vi "REPORT_OKNOK_save_pdf.vi"(8 "error_in":errorcluster) -> (0 "error_out":errorcluster)   [LabVIEW 2019]
uses:
  FGV/REPORTS_records_display/FGV_REPORTS_records_display.ctl
  typedef/REPORT_OKNOK_all_info.ctl
  <vilib>/Exaprom PDF/Controls/Table Controls/Row Predefined borders cluster.ctl
  <vilib>/Exaprom PDF/Controls/Table Controls/Row Predefined borders.ctl
  <vilib>/Exaprom PDF/Controls/Page Controls/Page setup.ctl
  <vilib>/Exaprom PDF/Controls/Page Controls/Page size.ctl
  <vilib>/Exaprom PDF/Controls/Page Controls/Page Orientation.ctl
  <vilib>/Exaprom PDF/Controls/Page Controls/Page Layout Custom.ctl
  <vilib>/Exaprom PDF/Controls/Page Controls/Page margins.ctl
  REPORT_font_for_pdf_report.ctl
  <vilib>/Exaprom PDF/Controls/Font Controls/Font size.ctl
  <vilib>/Exaprom PDF/Controls/Font Controls/Font color.ctl
  <vilib>/Exaprom PDF/Controls/Font Controls/Type and encoding.ctl
  <vilib>/Exaprom PDF/Controls/Text Controls/Unicode/Type and run direction.ctl
  <vilib>/Exaprom PDF/Controls/Table Controls/Cell Font, type, Alignment and LS V2.ctl
  <vilib>/Exaprom PDF/Controls/Table Controls/Cell Type, Alignment and LS.ctl
  <vilib>/Exaprom PDF/Controls/Table Controls/Cell Alignment 20px.ctl
  <vilib>/Exaprom PDF/Controls/Table Controls/Text vertical arrangement.ctl
  <vilib>/Exaprom PDF/Controls/Text Controls/Line spacing.ctl
  <vilib>/Exaprom PDF/Controls/Font Controls/Font complete cluster.ctl
  <vilib>/Exaprom PDF/Controls/Image Controls/Image alignment and position.ctl
  <vilib>/Exaprom PDF/Controls/Image Controls/Image aligment.ctl
  <vilib>/Exaprom PDF/Controls/Table Controls/Table properties.ctl
  <vilib>/Exaprom PDF/Controls/Table Controls/Table position.ctl
  _misc/AULocalize/SubVIs/Get Localized Phrase Compact Interface 0D.vi
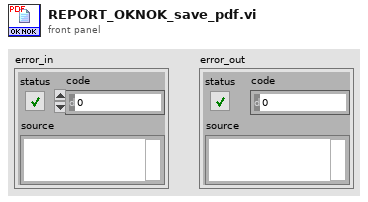
[diagram p1: front panel]
types:
  T1 = typedef "REPORT_OKNOK_all_info.ctl" = cluster{"date_start":string, "date_end":string, "time_start":string, "time_end":string, "records":string[][], "column_headers":string[], "column_widths":i16[]}
  T2 = typedef "FGV_REPORTS_records_display.ctl" = enum16{"initialize", "GEAR_set_serial", "GEAR_set_header", "GEAR_set_operations", "GEAR_set_results", "GEAR_set_batches", "GEAR_get_serial", "GEAR_get_operation_IDs", "GEAR_toggle_results", "GEAR_show_all_results", "GEAR_hide_all_results", "GEAR_display", "GEAR_filter", "GEAR_restore", "GEAR_clear", "GEAR_get_all_info", "DATES_set_dates", "DATES_set_gears", "DATES_display", "DATES_filter", "DATES_first_page", "DATES_previous_page", "DATES_next_page", "DATES_last_page", "DATES_restore", "DATES_clear", "DATES_get_all_info", "PBATCH_set_batch_no", "PBATCH_set_gears", "PBATCH_display", "PBATCH_filter", "PBATCH_first_page", "PBATCH_previous_page", "PBATCH_next_page", "PBATCH_last_page", "PBATCH_restore", "PBATCH_clear", "PBATCH_get_all_info", "OPRTN_set_OP", "OPRTN_set_dates", "OPRTN_set_gears", "OPRTN_set_hidden_columns", "OPRTN_display", "OPRTN_filter", "OPRTN_filter_no_page_reset", "OPRTN_first_page", "OPRTN_previous_page", "OPRTN_next_page", "OPRTN_last_page", "OPRTN_restore", "OPRTN_clear", "OPRTN_get_all_info", "CFG_set_type", "CFG_set_dates", "CFG_set_records", "CFG_display", "CFG_filter", "CFG_first_page", "CFG_previous_page", "CFG_next_page", "CFG_last_page", "CFG_restore", "CFG_clear", "CFG_get_all_info", "AUDIT_set_dates", "AUDIT_set_records", "AUDIT_display", "AUDIT_filter", "AUDIT_first_page", "AUDIT_previous_page", "AUDIT_next_page", "AUDIT_last_page", "AUDIT_restore", "AUDIT_clear", "AUDIT_get_all_info", "OKNOK_set_dates", "OKNOK_set_records", "OKNOK_display", "OKNOK_restore", "OKNOK_clear", "OKNOK_get_all_info", "REWORKS_set_dates", "REWORKS_set_from_to", "REWORKS_set_records", "REWORKS_display", "REWORKS_filter", "REWORKS_first_page", "REWORKS_previous_page", "REWORKS_next_page", "REWORKS_last_page", "REWORKS_restore", "REWORKS_clear", "REWORKS_get_all_info", "PACE_set_dates", "PACE_set_limits", "PACE_set_records", "PACE_display", "PACE_restore", "PACE_clear", "PACE_get_all_info", "CBATCH_set_code", "CBATCH_set_records", "CBATCH_display", "CBATCH_filter", "CBATCH_first_page", "CBATCH_previous_page", "CBATCH_next_page", "CBATCH_last_page", "CBATCH_restore", "CBATCH_clear", "CBATCH_get_all_info", "CMPNT_set_serial", "CMPNT_set_records", "CMPNT_display", "CMPNT_first_page", "CMPNT_previous_page", "CMPNT_next_page", "CMPNT_last_page", "CMPNT_restore", "CMPNT_clear", "CMPNT_get_all_info", "clear"}
  T3 = typedef "Table properties.ctl" = cluster{"Table position":T4, "SpacingBefore (points)":sgl, "SpacingAfter (points)":sgl}
  T4 = typedef "Table position.ctl" = i32
  T5 = typedef "Image alignment and position.ctl" = cluster{"Alignment":T6, "X ":sgl, "Y":sgl, "Indentation":sgl}
  T6 = typedef "Image aligment.ctl" = enum16{"Absolute (X,Y)", "Left", "Center", "Right", "Left (textwrap)", "Right (textwrap)"}
  T7 = typedef "Cell Font, type, Alignment and LS V2.ctl" = cluster{"Cell Type, Alignment and LS":T8, "Font":T12}
  T8 = typedef "Cell Type, Alignment and LS.ctl" = cluster{"Cell Alignment":T9, "Text rotation":T10, "Line spacing":T11}
  T9 = typedef "Cell Alignment 20px.ctl" = u16
  T10 = typedef "Text vertical arrangement.ctl" = enum16{"None", "Clockwise", "Counterclockwise"}
  T11 = typedef "Line spacing.ctl" = enum16{"Select", "1.0", "1.5", "2.0"}
  T12 = typedef "Font complete cluster.ctl" = cluster{"Name":string, "Size":T13, "Color":T14, "Style":cluster{"Bold":bool, "Italic":bool, "Underline":bool, "Strikeout":bool}, "Type":T15}
  T13 = typedef "Font size.ctl" = sgl
  T14 = typedef "Font color.ctl" = u32
  T15 = typedef "Type and encoding.ctl" = cluster{"Type&direction":T16, "Embedded":bool, "Encoding":string}
  T16 = typedef "Type and run direction.ctl" = enum16{"Select", "ASCII", "UTF-16", "UTF-16 (default)", "UTF-16 (LTR)", "UTF-16 (RTL)"}
  T17 = typedef "Page setup.ctl" = cluster{"Page Size":T18, "Orientation":T19, "Custom Size":T20, "Margins":T21}
  T18 = typedef "Page size.ctl" = i32
  T19 = typedef "Page Orientation.ctl" = enum16{"Portrait", "Landscape"}
  T20 = typedef "Page Layout Custom.ctl" = cluster{"Width":sgl, "Height":sgl}
  T21 = typedef "Page margins.ctl" = cluster{"Left":sgl, "Right":sgl, "Top":sgl, "Bottom":sgl}
  T22 = cluster{"Font Name:":string, "Size":i16, "Strikeout?":bool, "Italic?":bool, "Underline?":bool, "Outline?":bool, "Shadow?":bool, "Bold?":bool}
  T23 = typedef "Row Predefined borders cluster.ctl" = cluster{"Borders":T24, "Header":cluster{"Thickness":sgl, "Line":u32, "Background ":u32}, "Data":cluster{"Thickness":sgl, "Line":u32, "Background ":u32}}
  T24 = typedef "Row Predefined borders.ctl" = u16
  T25 = typedef "REPORT_font_for_pdf_report.ctl" = cluster{"Name":string, "Size":T13, "Color":T14, "Style":cluster{"Bold":bool, "Italic":bool, "Underline":bool, "Strikeout":bool}, "Type":T15}
  T26 = typedef "Table Appearance and Font Row [ ].ctl" = T27[]
  T27 = typedef "One Row Appearance.ctl" = cluster{"Row":T28, "Cell [ ]":T29[]}
  T28 = typedef "Row from to.ctl" = cluster{"From #":i16, "to #":i16}
  T29 = typedef "Cell, Alignment, LS and Font - hide Vmerge.ctl" = cluster{"Text":T8, "Cell Appearance":T30, "HMerge":T32, "VMerge":T33, "Font":T12}
  T30 = typedef "Cell Appearance.ctl" = cluster{"Border":T31, "Thickness":sgl, "Color":u32, "BG":u32}
  T31 = typedef "Cell Border 20 px.ctl" = u16
  T32 = typedef "Merge Horizontal.ctl" = cluster{"From":i8, "to":i8}
  T33 = typedef "Merge Vertical.ctl" = cluster{"From":i8, "to":i8}
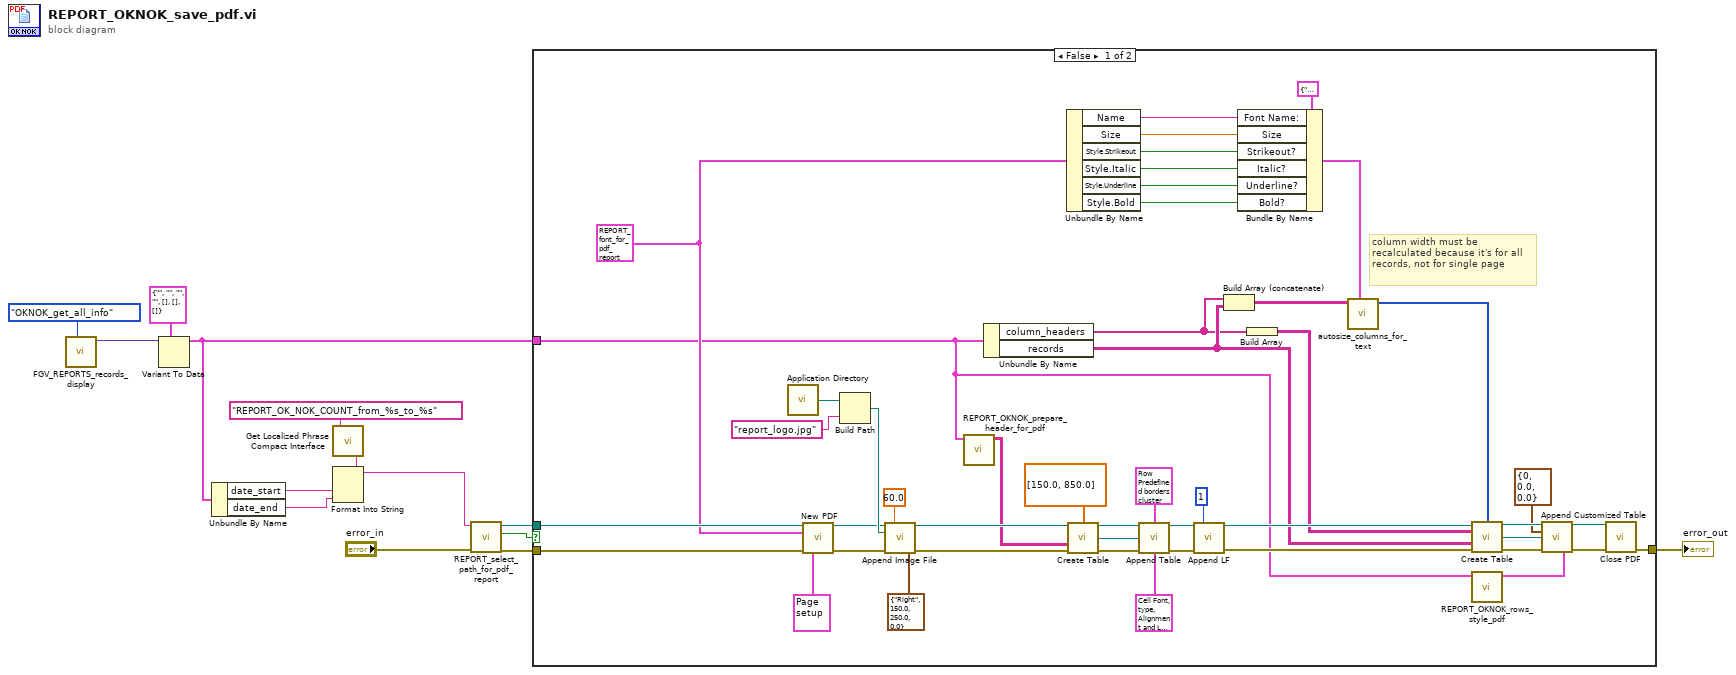
[diagram p0: block diagram]
diagram:
  n1 = call "FGV_REPORTS_records_display.vi"("options"=FGV_REPORTS_records_display."OKNOK_get_all_info") -> ("output"=w14:variant)  [unwired: 9 in, 1 out]
  n2 = Variant To Data(type=T1 {"date_start"="", "date_end"="", "time_start"="", "time_end"="", "records"=[], "column_headers"=[], "column_widths"=[]} ("REPORT_OKNOK_all_info"), Variant=w14) -> (data=w3:T1)  [unwired: 1 in, 1 out]
  n3 = Unbundle By Name(w3) -> ("date_start"=w7:string, "date_end"=w5:string)
  n4 = call-poly "Get Localized Phrase Compact Interface.vi"("Key"="REPORT_OK_NOK_COUNT_from_%s_to_%s" ("report_title")) -> ("Translated Phrase"=w1:string)
  n5 = Format Into String(format string=w1, w7, w5) -> (resulting string=w6:string)  [unwired: 2 in, 1 out]
  n6 = call "REPORT_select_path_for_pdf_report.vi"("error_in"="error_in", "report_title"=w6) -> ("error_out"=w9:errorcluster, "cancelled"=w2:bool, "path_to_report"=w10:path)  [unwired: 7 in]
  n7 = case shown="False" w2 {
    tunnel: [w61 w62] -> w11
    tunnel: w10 -> [w60 _]
    tunnel: w9 -> [w59 w62]
    tunnel: w3 -> [w16 _]
    frame False {
      w25 = T25 {"Name"="Consolas", "Size"=10.0, "Color"=0, "Style"={"Bold"=FALSE, "Italic"=FALSE, "Underline"=FALSE, "Strikeout"=FALSE}, "Type"={"Type&direction"=enum."ASCII", "Embedded"=FALSE, "Encoding"="CP855"}} ("Default Font")
      # "column width must be recalculated because it's for all records, not for single page"
      n8 = call <vilib>:"Application Directory.vi"() -> ("Application Directory"=w53:path)
      n9 = call <vilib>:"New PDF.vi"("PDF Path"=w60, "Default Font"=w25, "error in (no error)"=w59, "Page Setup"=T17 {"Page Size"=11, "Orientation"=enum."Landscape", "Custom Size"={"Width"=216.0, "Height"=279.0}, "Margins"={"Left"=10.0, "Right"=10.0, "Top"=10.0, "Bottom"=10.0}}) -> ("PDF Report"=w47:refnum<class "PDF Report Class.lvclass">, "error out"=w48:errorcluster)  [unwired: 7 in, 3 out]
      n10 = Build Path(base path=w53, name or relative path="report_logo.jpg") -> (appended path=w49:path)
      n11 = call <vilib>:"Append Image File.vi"("PDF Report IN"=w47, "Scale (%)"=sgl 60.0, "Image path"=w49, "error in (no error)"=w48, "Position and indentation"=T5 {"Alignment"=enum."Right", "X "=150.0, "Y"=250.0, "Indentation"=0.0}) -> ("PDF Report OUT"=w32:refnum<class "PDF Report Class.lvclass">, "error out"=w31:errorcluster)  [unwired: 7 in, 2 out]
      n12 = call "REPORT_OKNOK_prepare_header_for_pdf.vi"("REPORT_OKNOK_all_info"=w16) -> ("report_header"=w30:string[][])  [unwired: 10 in]
      n13 = Unbundle By Name(w16) -> ("column_headers"=w28:string[], "records"=w29:string[][])
      n14 = Unbundle By Name(w25) -> ("Name"=w22:string, "Size"=w21:T13, "Style.Strikeout"=w20:bool, "Style.Italic"=w19:bool, "Style.Underline"=w18:bool, "Style.Bold"=w17:bool)
      n15 = call <vilib>:"Create Table.vi"("PDF Report IN"=w32, "Table columnWidth [ ]"=sgl[] [150.0, 850.0], "Text Data 2D [ ]"=w30, "error in (no error)"=w31) -> ("PDF Report duplicate"=w40:refnum<class "PDF Report Class.lvclass">, "PDF Table"=w39:refnum<class "Pdfp Table Class.lvclass">, "error out"=w38:errorcluster)  [unwired: 9 in]
      n16 = call <vilib>:"Append Table.vi"("PDF Report IN"=w40, "Predefined Borders"=T23 {"Borders"=0, "Header"={"Thickness"=0.0, "Line"=0, "Background "=16777215}, "Data"={"Thickness"=0.0, "Line"=0, "Background "=16777215}}, "PDF Table"=w39, "error in (no error)"=w38, "Datas format"=T7 {"Cell Type, Alignment and LS"={"Cell Alignment"=0, "Text rotation"=enum."None", "Line spacing"=enum."Select"}, "Font"={"Name"="Consolas", "Size"=-1.0, "Color"=0, "Style"={"Bold"=FALSE, "Italic"=FALSE, "Underline"=FALSE, "Strikeout"=FALSE}, "Type"={"Type&direction"=enum."Select", "Embedded"=FALSE, "Encoding"=""}}}) -> ("PDF Report OUT"=w37:refnum<class "PDF Report Class.lvclass">, "error out"=w36:errorcluster)  [unwired: 9 in]
      n17 = call <vilib>:"Append LF.vi"("PDF Report IN"=w37, "Number of LF (default 1)"=u8 1, "error in (no error)"=w36) -> ("PDF Report duplicate"=w45:refnum<class "PDF Report Class.lvclass">, "error out"=w44:errorcluster)  [unwired: 11 in]
      n18 = Build Array (concatenate)(w28, w29) -> (w27:string[][])
      n19 = Bundle By Name(cluster=T22 {"Font Name:"="", "Size"=0, "Strikeout?"=FALSE, "Italic?"=FALSE, "Underline?"=FALSE, "Outline?"=FALSE, "Shadow?"=FALSE, "Bold?"=FALSE} ("font"), "Font Name:"=w22, "Size"=w21, "Strikeout?"=w20, "Italic?"=w19, "Underline?"=w18, "Bold?"=w17) -> (w24:T22)
      n20 = Build Array(w28) -> (w42:string[][])
      n21 = call "autosize_columns_for_text.vi"("font"=w24, "array_to_autosize"=w27) -> ("column_widths"=w26:i16[])  [unwired: 9 in]
      n22 = call <vilib>:"Create Table.vi"("PDF Report IN"=w45, "Table columnWidth [ ]"=w26, "Column Headers 2D [ ]"=w42, "Text Data 2D [ ]"=w29, "error in (no error)"=w44) -> ("PDF Report duplicate"=w43:refnum<class "PDF Report Class.lvclass">, "PDF Table"=w55:refnum<class "Pdfp Table Class.lvclass">, "error out"=w58:errorcluster)  [unwired: 8 in]
      n23 = call "REPORT_OKNOK_rows_style_pdf.vi"("REPORT_OKNOK_all_info"=w16) -> ("Row  [ ]"=w41:T26)  [unwired: 10 in]
      n24 = call <vilib>:"Append Customized Table.vi"("PDF Report IN"=w43, "Table properties"=T3 {"Table position"=0, "SpacingBefore (points)"=0.0, "SpacingAfter (points)"=0.0}, "PDF Table"=w55, "error in (no error)"=w58, "Row  [ ]"=w41) -> ("PDF Report OUT"=w56:refnum<class "PDF Report Class.lvclass">, "error out"=w57:errorcluster)  [unwired: 9 in]
      n25 = call <vilib>:"Close PDF.vi"("PDF Report"=w56, "error in (no error)"=w57) -> ("error out"=w61:errorcluster)  [unwired: 12 in, 1 out]
    }
    frame True {
    }
  }
  "error_out" <- w11
